vi "HEWH Power Off Check.vi"(0 "input cluster":T1, 7 "Init":bool, 11 "Heating off Time(s)":dbl=5.0) -> (4 "Heat turn off time":dbl, 8 "Heat Off, Really":bool)   [LabVIEW 2014]
uses:
  Type Definitions/HEWH Power Elements.ctl
panel:
  out "Elapsed Time (sec)":dbl format="%.2f"
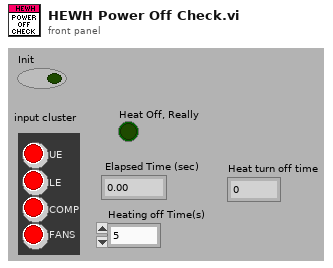
[diagram p1: front panel]
types:
  T1 = typedef "HEWH Power Elements.ctl" = cluster{"UE":bool, "LE":bool, "COMP":bool, "FANS":bool}
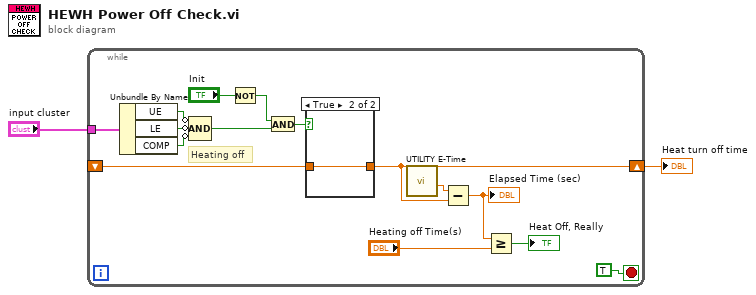
[diagram p0: block diagram]
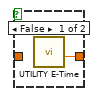
[diagram p2: hidden frame]
diagram:
  n1 = while {
    tunnel: "input cluster" -> [w14]
    shift-right: [w10] -> w1
    shift-left: _ -> [w12]
    stop <- TRUE stop-if-true
    # "Heating off"
    n2 = Unbundle By Name(w14) -> ("UE"=w15:bool, "LE"=w17:bool, "COMP"=w16:bool)
    n3 = Compound Arithmetic op=AND(invert w15, invert w17, invert w16) -> (w13:bool)
    n4 = Not(x="Init") -> (.not. x?=w7:bool)
    n5 = And(x=w7, y=w13) -> (x .and. y?=w9:bool)
    n6 = case shown="True" w9 {
      tunnel: [w18 w19] -> w10
      tunnel: w12 -> [_ w19]
      frame False {
        n7 = call "UTILITY E-Time.vi"() -> ("Elapsed Time (sec)"=w18:dbl)  [unwired: 9 in, 2 out]
      }
      frame True {
      }
    }
    n8 = call "UTILITY E-Time.vi"() -> ("Elapsed Time (sec)"=w11:dbl)  [unwired: 9 in, 2 out]
    n9 = Subtract(x=w11, y=w10) -> (x-y=w3:dbl)
    "Elapsed Time (sec)" <- w3
    n10 = Greater Or Equal?(x=w3, y="Heating off Time(s)") -> (x >= y?=→"Heat Off, Really":bool)
  }
  "Heat turn off time" <- w1
